vi "send message.vi"(5 "mask? (F)":bool, 6 "timeout ms (5000)":i32=5000, 7 "final fragment (T)":bool=TRUE, 8 "error in":errorcluster, 9 "opcode":u8, 10 "data":string, 11 "TCP Network Connection in":refnum<k5>) -> (0 "error out":errorcluster)   [LabVIEW 2013, in "websocket core.lvlib"]
uses:
  websocket core.lvlib
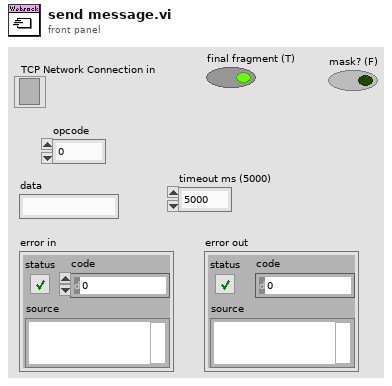
[diagram p1: front panel]
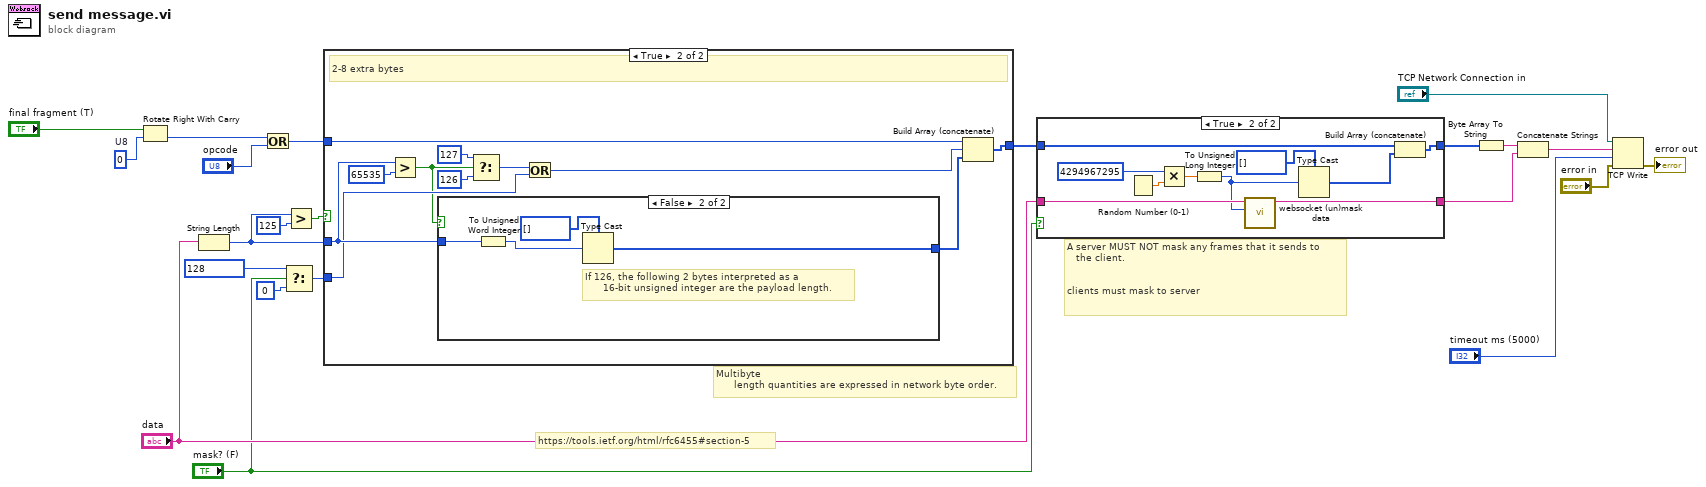
[diagram p0: block diagram]
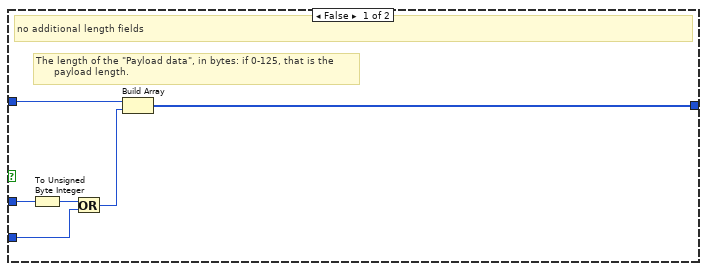
[diagram p3: hidden frame]
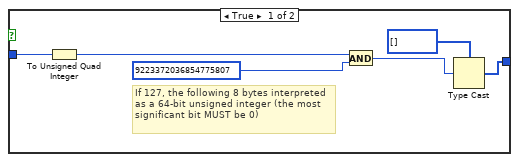
[diagram p4: hidden frame]
diagram:
  w13 = u8 0  # U8
  # "https://tools.ietf.org/html/rfc6455#section-5"
  # "Multibyte\n      length quantities are expressed in network byte order."
  # "A server MUST NOT mask any frames that it sends to\n   the client.\n\n\nclients must mask to server"
  n1 = Rotate Right With Carry(2:w13, 3:"final fragment (T)") -> (0:w12:u8)  [unwired: 1 out]
  n2 = String Length(string="data") -> (length=w18:i32)
  n3 = Or(x=w12, y="opcode") -> (x .or. y?=w19:u8)
  n4 = Select(t=u8 128 ("x"), s="mask? (F)", f=u8 0 ("x")) -> (s? t:f=w4:u8)
  n5 = Greater?(x=w18, y=125 ("upper limit")) -> (0:w15:bool)
  n6 = case shown="True" w15 {
    tunnel: w18 -> [w28 w38]
    tunnel: [w23 w30] -> w1
    tunnel: w19 -> [w25 w33]
    tunnel: w4 -> [w26 w35]
    frame False {
      # "The length of the \"Payload data\", in bytes: if 0-125, that is the\n      payload length."
      # "no additional length fields"
      n7 = To Unsigned Byte Integer(number=w28) -> (unsigned 8bit integer=w27:u8)
      n8 = Or(x=w27, y=w26) -> (x .or. y?=w24:u8)
      n9 = Build Array(w25, w24) -> (w23:u8[])
    }
    frame True {
      # "2-8 extra bytes"
      n10 = Greater?(x=w38, y=65535) -> (0:w29:bool)
      n11 = case shown="False" w29 {
        tunnel: w38 -> [w45 w49]
        tunnel: [w42 w46] -> w31
        frame True {
          # "If 127, the following 8 bytes interpreted as a 64-bit unsigned integer (the most significant bit MUST be 0)"
          n12 = To Unsigned Quad Integer(1:w45) -> (0:w44:u64)
          n13 = And(x=w44, y=u64 9223372036854775807 ("unsigned 64bit integer")) -> (x .and. y?=w41:u64)
          n14 = Type Cast(type=u8[] [], x=w41) -> (*(type *) &x=w42:u8[])
        }
        frame False {
          # "If 126, the following 2 bytes interpreted as a\n      16-bit unsigned integer are the payload length."
          n15 = To Unsigned Word Integer(number=w49) -> (unsigned 16bit integer=w48:u16)
          n16 = Type Cast(type=u8[] [], x=w48) -> (*(type *) &x=w46:u8[])
        }
      }
      n17 = Select(t=u8 127 ("U8"), s=w29, f=u8 126 ("U8")) -> (s? t:f=w36:u8)
      n18 = Or(x=w36, y=w35) -> (x .or. y?=w32:u8)
      n19 = Build Array (concatenate)(w33, w32, w31) -> (w30:u8[])
    }
  }
  n20 = case shown="True" "mask? (F)" {
    tunnel: [w51 w60] -> w8
    tunnel: "data" -> [w51 w61]
    tunnel: [w50 w55] -> w2
    tunnel: w1 -> [w50 w56]
    frame False {
    }
    frame True {
      n21 = Random Number (0-1)() -> (number: 0 to 1=w59:dbl)
      n22 = Multiply(x=u32 4294967295, y=w59) -> (x*y=w57:dbl)
      n23 = To Unsigned Long Integer(number=w57) -> (unsigned 32bit integer=w53:u32)
      n24 = call "websocket (un)mask data.vi"("mask key"=w53, "masked data"=w61) -> ("unmasked data"=w60:string)  [unwired: 9 in]
      n25 = Type Cast(type=u8[] [], x=w53) -> (*(type *) &x=w52:u8[])
      n26 = Build Array (concatenate)(w56, w52) -> (w55:u8[])
    }
  }
  n27 = Byte Array To String(unsigned byte array=w2) -> (string=w17:string)
  n28 = Concatenate Strings(w17, w8) -> (w16:string)
  n29 = TCP Write(connection ID="TCP Network Connection in", data in=w16, error in (no error)="error in", 9:"timeout ms (5000)") -> (error out=→"error out":errorcluster)  [unwired: 2 out]
